vi "FindFRF.vi"(2 "Microphone FFT":cluster{dbl, "df":dbl, "FFT {X}":cdb[]}, 3 "Hammer FFT":cluster{dbl, "df":dbl, "FFT {X}":cdb[]}) -> (0 "Coherence":cluster{dbl, "df":dbl, dbl[]}(graph), 1 "Current FRF":cluster{dbl, "df":dbl, dbl[]}(graph))   [LabVIEW 2014]
panel:
  out "All Info":cluster{dbl, "df":dbl, dbl[]}[](graph)=[{0.0, "df"=3.3349544917668315, array[8192 elements]}, {0.0, "df"=3.3349544917668315, array[8192 elements]}, {0.0, "df"=3.3349544917668315, array[8192 elements]}, {0.0, "df"=3.3349544917668315, array[8192 elements]}]
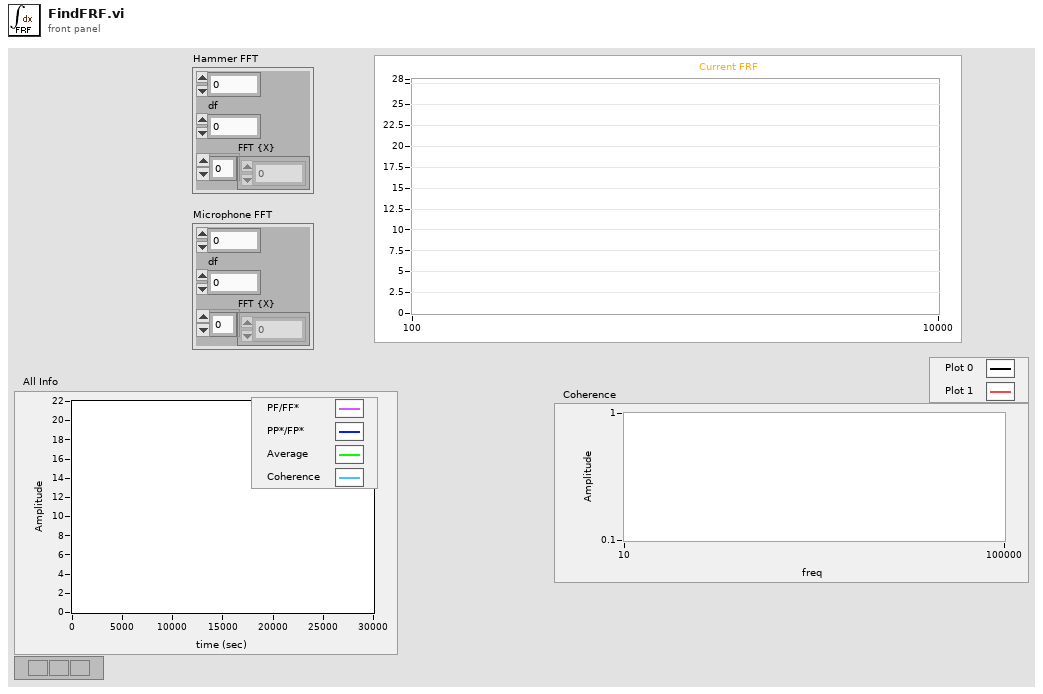
[diagram p1: front panel]
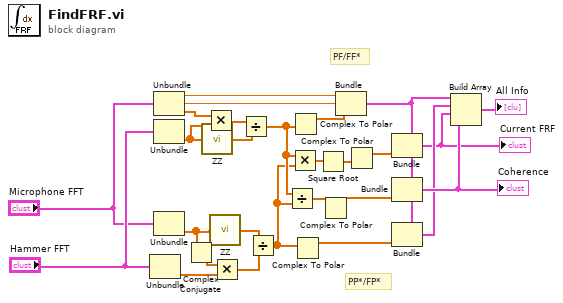
[diagram p0: block diagram]
diagram:
  # "PP*/FP*"
  # "PF/FF*"
  n1 = Unbundle("Hammer FFT") -> ("FFT {X}"=w24:cdb[])  [unwired: 2 out]
  n2 = Unbundle("Microphone FFT") -> (w19:dbl, "df"=w18:dbl, "FFT {X}"=w26:cdb[])
  n3 = Unbundle("Hammer FFT") -> ("FFT {X}"=w22:cdb[])  [unwired: 2 out]
  n4 = Unbundle("Microphone FFT") -> ("FFT {X}"=w17:cdb[])  [unwired: 2 out]
  n5 = Complex Conjugate(1:w17) -> (0:w16:cdb[])
  n6 = call <userlib>:"ZZ.vi"("P"=w22) -> ("PP*"=w21:dbl[])
  n7 = Multiply(x=w26, y=w22) -> (x*y=w23:cdb[])
  n8 = call <userlib>:"ZZ.vi"("P"=w17) -> ("PP*"=w20:dbl[])
  n9 = Multiply(x=w16, y=w24) -> (x*y=w25:cdb[])
  n10 = Divide(x=w23, y=w21) -> (x/y=w11:cdb[])
  n11 = Divide(x=w20, y=w25) -> (x/y=w10:cdb[])
  n12 = Divide(x=w11, y=w10) -> (x/y=w13:cdb[])
  n13 = Multiply(x=w11, y=w10) -> (x*y=w9:cdb[])
  n14 = Complex To Polar(r * e^(i*theta)=w11) -> (r=w15:dbl[])  [unwired: 1 out]
  n15 = Complex To Polar(r * e^(i*theta)=w10) -> (r=w14:dbl[])  [unwired: 1 out]
  n16 = Square Root(x=w9) -> (sqrt(x)=w8:cdb[])
  n17 = Complex To Polar(r * e^(i*theta)=w13) -> (r=w12:dbl[])  [unwired: 1 out]
  n18 = Bundle(w19, "df"=w18, w15) -> (w6:cluster{dbl, "df":dbl, dbl[]})  [unwired: 1 in]
  n19 = Complex To Polar(r * e^(i*theta)=w8) -> (r=w7:dbl[])  [unwired: 1 out]
  n20 = Bundle(cluster=w6, w7) -> (w1:cluster{dbl, "df":dbl, dbl[]})  [unwired: 2 in]
  "Current FRF" <- w1
  n21 = Bundle(cluster=w6, w12) -> (w27:cluster{dbl, "df":dbl, dbl[]})  [unwired: 2 in]
  "Coherence" <- w27
  n22 = Bundle(cluster=w6, w14) -> (w5:cluster{dbl, "df":dbl, dbl[]})  [unwired: 2 in]
  n23 = Build Array(w6, w5, w1, w27) -> (→"All Info":cluster{dbl, "df":dbl, dbl[]}[])
